vi "checkStatus.vi"(8 "error in (no error)":errorcluster, 10 "stop":bool, 11 "NetworkPixelfly in":refnum<class "NetworkPixelfly.lvclass">) -> (0 "error out":errorcluster, 2 "stopped?":bool, 3 "NetworkPixelfly out":refnum<class "NetworkPixelfly.lvclass">)   [LabVIEW 2011, in "Hardware.lvlib" / "HWControllers.lvlib" / "NetworkPixelfly.lvclass"]
uses:
  NetworkPixelfly.lvclass
  NetworkPixelfly.lvclass/NetworkPixelfly.ctl
  Channels/Channels.lvlib
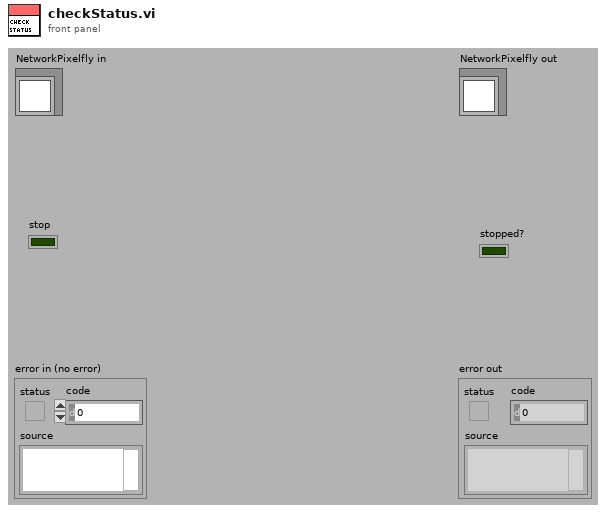
[diagram p1: front panel]
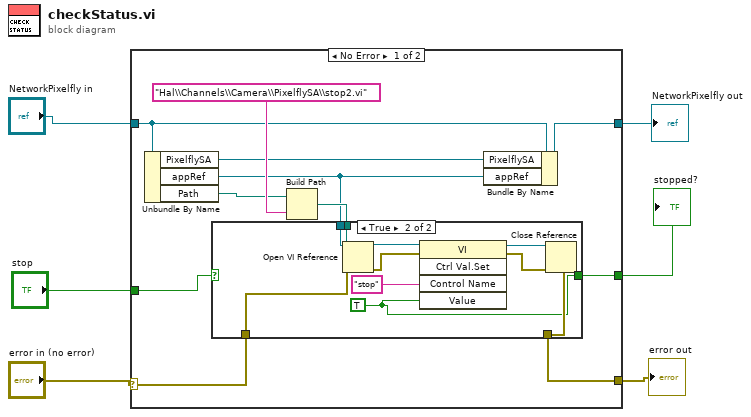
[diagram p0: block diagram]
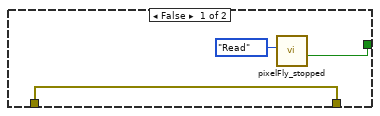
[diagram p2: hidden frame]
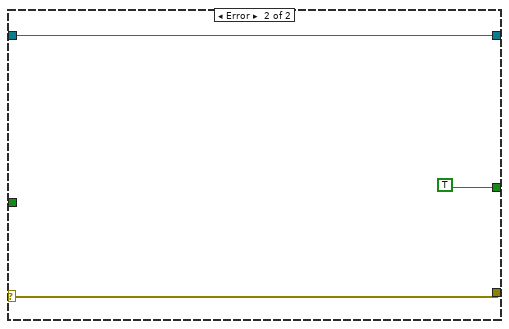
[diagram p3: hidden frame]
diagram:
  n1 = case shown="No Error" "error in (no error)" {
    selector: "error in (no error)" -> [w15 w32]
    tunnel: [w9 w32] -> w6
    tunnel: "NetworkPixelfly in" -> [w11 w33]
    tunnel: [w10 w33] -> w4
    tunnel: "stop" -> [w8 _]
    tunnel: [w13 TRUE] -> w1
    frame No Error {
      n2 = Unbundle By Name(w11) -> ("PixelflySA"=w7:refnum<class "PixelflySA.lvclass">, "appRef"=w12:refnum<vi>, "Path"=w14:path)
      n3 = Build Path(base path=w14, name or relative path="Hal\\Channels\\Camera\\PixelflySA\\stop2.vi") -> (appended path=w16:path)
      n4 = case shown="True" w8 {
        tunnel: w16 -> [_ w30]
        tunnel: w15 -> [w18 w29]
        tunnel: [w19 w21] -> w13
        tunnel: w12 -> [_ w28]
        tunnel: [w18 w27] -> w9
        frame False {
          n5 = call "pixelFly_stopped.vi"("Action"=enum16{"Write", "Read"}."Read") -> ("stopped"=w19:bool)  [unwired: 10 in]
        }
        frame True {
          w21 = TRUE
          n6 = Open VI Reference(application reference (local)=w28, vi path=w30, error in (no error)=w29) -> (vi reference=w25:refnum<vi>, error out=w26:errorcluster)  [unwired: 3 in]
          n7 = invoke class="VI" method="Ctrl Val.Set"(reference=w25, error in=w26, "Control Name"="stop", "Value"=w21) -> (reference out=w24:refnum<vi>, error out=w23:errorcluster)  [unwired: 1 in, 3 out]
          n8 = Close Reference(reference=w24, error in (no error)=w23) -> (error out=w27:errorcluster)
        }
      }
      n9 = Bundle By Name(cluster=w11, "PixelflySA"=w7, "appRef"=w12) -> (w10:refnum<class "NetworkPixelfly.lvclass">)
    }
    frame Error {
    }
  }
  "error out" <- w6
  "NetworkPixelfly out" <- w4
  "stopped?" <- w1
